vi "11115 UI.vi"(8 "error in (no error)":errorcluster, 11 "Node Ptr":T1 format="%.0x") -> (0 "error out":errorcluster)   [LabVIEW 2019, in "Modules.lvlib" / "11115.lvclass"]
uses:
  11115.lvclass
  <vilib>/NI VeriStand/Custom Device API/Custom Device Item Ref.ctl
  RSI Module/SubPanel Command.ctl
  C:/Users/nitest/Desktop/Git 2019/niveristand-scan-engine-module-libraries/Source/RemIO Module/RemIO Module.lvclass
  11115.lvclass/11115.ctl
  <vilib>/indcomecat/Remote IO/typedefs/REM-11115/channel number REM-11115.ctl
  RemIO Module/RemIO Module.lvclass
  <vilib>/indcomecat/Remote IO/NI ECAT Remote IO.lvlib
  <vilib>/NI VeriStand/Custom Device API/Custom Device API.lvlib
  RSI Module/RSI Module.lvclass
panel:
  in  "Output Range":u8[](array[ring])=[0, 0, 0, 0] items=["0 V ... 10 V"=0, "-10 V ... 10 V"=1, "0 V ... 5 V"=2, "-5 V ... 5V"=3, "0 mA ... 20 mA"=4, "4 mA ... 20 mA"=6, "Channel inactive"=15]
  out "_Chan0Label":string="Channel 0"
  out "_Chan1Label":string="Channel 1"
  out "_Chan2Label":string="Channel 2"
  out "_Chan3Label":string="Channel 3"
  out "_Outputlabel":string="Output Range"
  in  "SubPanel Event":refnum<user-event>
  in  "Header":cluster{"Section Name":string}={"Section Name"="NI REM-11115 Settings"}
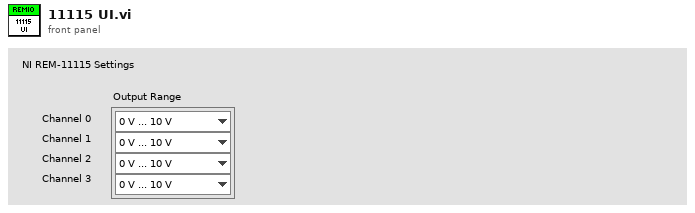
[diagram p1: front panel]
types:
  T1 = typedef "Custom Device API.lvlib/Custom Device Item Ref.ctl" = u64
  T2 = typedef "NI ECAT Remote IO.lvlib/channel number REM-11115.ctl" = u8
  T3 = typedef "NI ECAT Remote IO.lvlib/output range REM-11115.ctl" = u8
  T4 = cluster{"channel number":T2, "output range":T3}[]
  T5 = typedef "Modules.lvlib/RSI Module.lvclass/SubPanel Command.ctl" = enum16{"Stop"}
  T6 = cluster{"channel number":T2, "Output Range 3":u8}
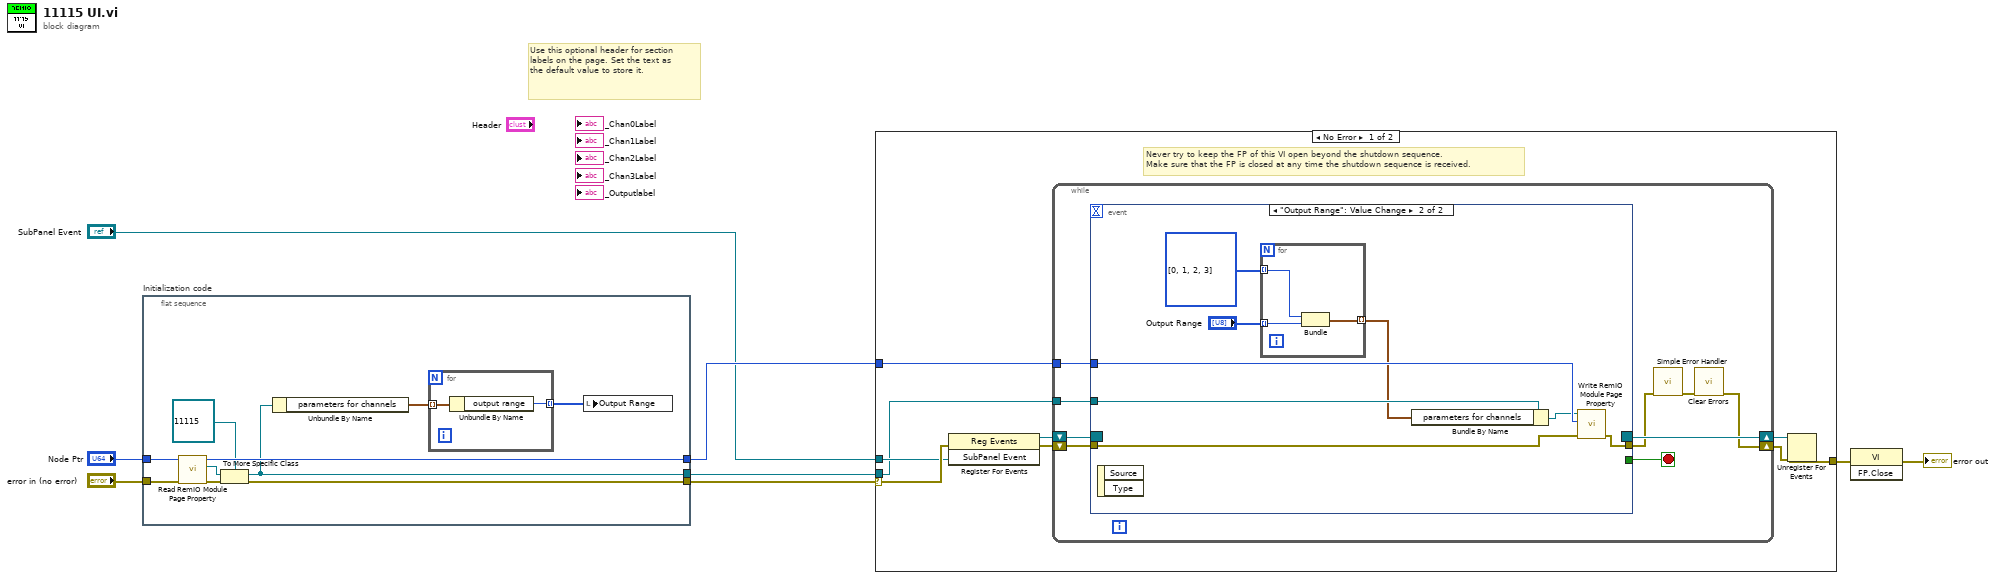
[diagram p0: block diagram]
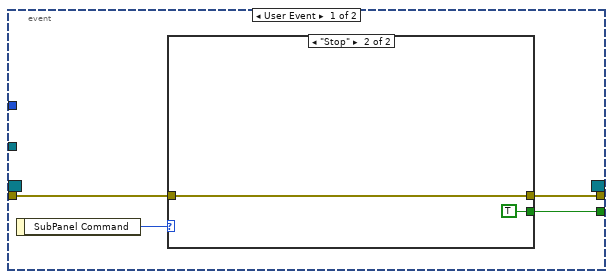
[diagram p2: hidden frame]
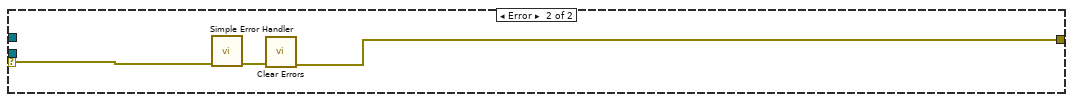
[diagram p4: hidden frame]
diagram:
  # "Use this optional header for section labels on the page. Set the text as the default value to store it."
  n1 = flat-sequence "Initialization code" {
    tunnel: "error in (no error)" -> [w17]
    tunnel: "Node Ptr" -> [w18]
    tunnel: [w13] -> w2
    tunnel: [w16] -> w5
    tunnel: [w11] -> w1
    frame #0 {
      n2 = call "Read RemIO Module Page Property.vi"("error in (no error)"=w17, "Node Ptr In"=w18) -> ("error out"=w15:errorcluster, "RemIO Module"=w14:refnum<class "RemIO Module.lvclass">, "Node Ptr Out"=w16:T1)  [unwired: 7 in]
      n3 = To More Specific Class(target class=refnum<class "11115.lvclass"> refnum ("Modules.lvlib:11115.lvclass"), reference=w14, error in=w15) -> (specific class reference=w11:refnum<class "11115.lvclass">, error out=w13:errorcluster)
      n4 = Unbundle By Name(w11) -> ("parameters for channels"=w10:T4)
      n5 = for {
        tunnel: w10 -> [w20] mode=indexing
        tunnel: [w19] -> w9 mode=indexing
        n6 = Unbundle By Name(w20) -> ("output range"=w19:T3)
      }
      n7 = local write "Output Range"(w9) -> ()
    }
  }
  n8 = case shown="No Error" w2 {
    selector: w2 -> [w23 w59]
    tunnel: [w27 w57] -> w8
    tunnel: w5 -> [w24 _]
    tunnel: "SubPanel Event" -> [w22 _]
    tunnel: w1 -> [w21 _]
    frame No Error {
      # "Never try to keep the FP of this VI open beyond the shutdown sequence.\nMake sure that the FP is closed at any time the shutdown sequence is received."
      n9 = register-events(error in=w23, w22) -> (reference out=w25:refnum<event-registration>, error out=w26:errorcluster)  [unwired: 1 in]
      n10 = while {
        tunnel: w24 -> [w34]
        shift-right: [w31] -> w28
        shift-left: w26 -> [w37]
        shift-right: [w38] -> w29
        shift-left: w25 -> [w36]
        tunnel: w21 -> [w30]
        stop <- w35 stop-if-true
        n11 = event shown="[1] \"Output Range\": Value Change" {
          selector: w36 -> [_ _]
          dyn-events: [_ _] -> w38
          timeout: _ -> [_ _]
          tunnel: w37 -> [w41 w51]
          tunnel: [w39 _] -> w35
          tunnel: [w40 w50] -> w33
          tunnel: w34 -> [_ w52]
          tunnel: w30 -> [_ w53]
          event User Event {
            n12 = event-data() -> ("SubPanel Command"=w42:T5)  [unwired: 1 out]
            n13 = case shown="\"Stop\"" w42 {
              tunnel: w41 -> [w43 w44]
              tunnel: [w43 w44] -> w40
              tunnel: [_ TRUE] -> w39
              frame Default {
              }
              frame "Stop" {
              }
            }
          }
          event "Output Range": Value Change {
            w47 = T2[] [0, 1, 2, 3] items=["AO0", "AO1", "AO2", "AO3"]
            n14 = event-data() -> ()  [unwired: 3 out]
            n15 = for {
              tunnel: "Output Range" -> [w56] mode=indexing
              tunnel: w47 -> [w54] mode=indexing
              tunnel: [w55] -> w46 mode=indexing
              n16 = Bundle("channel number"=w54, "Output Range 3"=w56) -> (w55:T6)  [unwired: 1 in]
            }
            n17 = Bundle By Name(cluster=w53, "parameters for channels"=w46) -> (w49:refnum<class "11115.lvclass">)
            n18 = call "Write RemIO Module Page Property.vi"("error in (no error)"=w51, "Node Ptr In"=w52, "RemIO Module"=w49) -> ("error out"=w50:errorcluster)  [unwired: 6 in, 2 out]
          }
        }
        n19 = call <vilib>:"Simple Error Handler.vi"("error in (no error)"=w33) -> ("error out"=w32:errorcluster)  [unwired: 1 in, 7 out]
        n20 = call <vilib>:"Clear Errors.vi"("error in (no error)"=w32) -> ("error out"=w31:errorcluster)  [unwired: 1 in, 5 out]
      }
      n21 = Unregister For Events(event registration refnum=w29, error in=w28) -> (error out=w27:errorcluster)
    }
    frame Error {
      n22 = call <vilib>:"Simple Error Handler.vi"("error in (no error)"=w59) -> ("error out"=w58:errorcluster)  [unwired: 1 in, 7 out]
      n23 = call <vilib>:"Clear Errors.vi"("error in (no error)"=w58) -> ("error out"=w57:errorcluster)  [unwired: 1 in, 5 out]
    }
  }
  n24 = invoke class="VI" method="FP.Close"(error in=w8) -> (error out=→"error out":errorcluster)  [unwired: 2 in, 2 out]
